vi "IBM4_Open.vi"(11 "COM Port":refnum<visa-resource-name>="COM3") -> (0 "error out":errorcluster, 2 "UCC Revision #":string, 3 "COM resource out":refnum<visa-resource-name>)   [LabVIEW 2021, in "IBM4.lvlib"]
doc: "Open the IBM4"
uses:
  <instrlib>/IBM4/IBM4.lvlib
  <vilib>/Instr/_visa.llb/VISA Configure Serial Port (Instr).vi
panel:
  out "read buffer":string
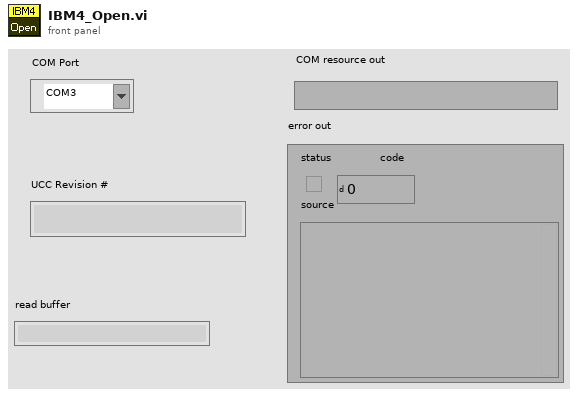
[diagram p1: front panel]
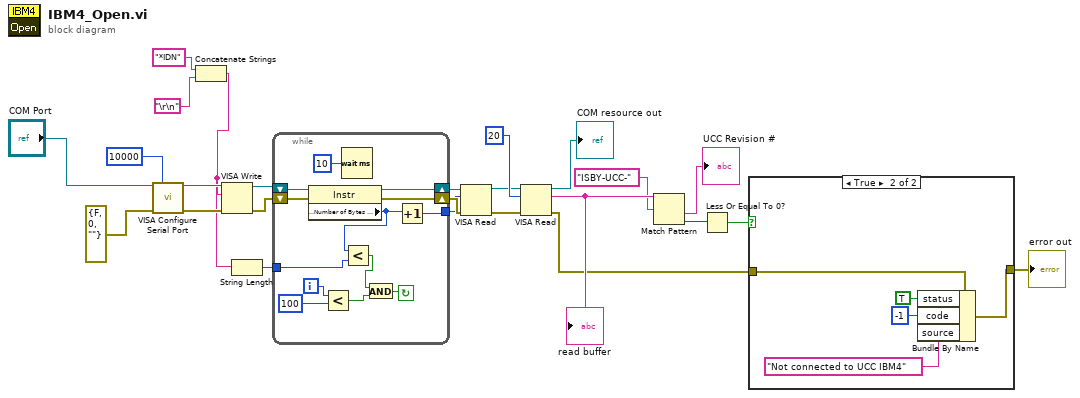
[diagram p0: block diagram]
diagram:
  n1 = call-poly "VISA Configure Serial Port"("VISA resource name"="COM Port", "timeout (10sec)"=u32 10000, "error in (no error)"=errorcluster {"status"=FALSE, "code"=0, "source"=""}) -> ("VISA resource name out"=w22:refnum<visa-resource-name>, "error out"=w21:errorcluster)  [unwired: 11 in]
  n2 = Concatenate Strings("*IDN" ("write buffer"), "\r\n") -> (w9:string)
  n3 = VISA Write(VISA resource name=w22, write buffer=w9, error in (no error)=w21) -> (VISA resource name out=w16:refnum<visa-resource-name>, error out=w15:errorcluster)  [unwired: 1 out]
  n4 = String Length(string=w9) -> (length=w8:i32)
  n5 = while {
    tunnel: [w27] -> w12
    shift-right: [w37] -> w14
    shift-left: w16 -> [w38]
    shift-right: [w35] -> w13
    shift-left: w15 -> [w36]
    tunnel: w8 -> [w33]
    i -> [w28]
    stop <- w31 continue-if-true
    n6 = property class="Instr"(reference=w38, error in=w36) -> (reference out=w37:refnum<visa-resource-name>, error out=w35:errorcluster, "Serial Settings:Number of Bytes at Serial Port"=w26:u32)
    n7 = Less?(x=w28, y=100) -> (x < y?=w30:bool)
    n8 = Wait (ms)(milliseconds to wait=u32 10) -> ()  [unwired: 1 out]
    n9 = Less?(x=w26, y=w33) -> (x < y?=w29:bool)
    n10 = And(x=w29, y=w30) -> (x .and. y?=w31:bool)
    n11 = Increment(x=w26) -> (x+1=w27:u32)
  }
  n12 = VISA Read(VISA resource name=w14, byte count=w12, error in (no error)=w13) -> (VISA resource name out=w11:refnum<visa-resource-name>, error out=w10:errorcluster)  [unwired: 2 out]
  n13 = VISA Read(VISA resource name=w11, byte count=u32 20, error in (no error)=w10) -> (VISA resource name out=→"COM resource out":refnum<visa-resource-name>, read buffer=w7:string, error out=w3:errorcluster)  [unwired: 1 out]
  "read buffer" <- w7
  n14 = Match Pattern(string=w7, regular expression="ISBY-UCC-" ("format string")) -> (after substring=→"UCC Revision #":string, offset past match=w4:i32)  [unwired: 1 in, 2 out]
  n15 = Less Or Equal To 0?(x=w4) -> (x <= 0?=w2:bool)
  n16 = case shown="True" w2 {
    tunnel: w3 -> [w39 w42]
    tunnel: [w39 w43] -> w1
    frame False {
    }
    frame True {
      n17 = Bundle By Name(cluster=w42, "status"=TRUE, "code"=-1, "source"="Not connected to UCC IBM4") -> (w43:errorcluster)
    }
  }
  "error out" <- w1
